vi "DestroyQ.vi"(8 "error in (no error)":errorcluster) -> (0 "error out":errorcluster)   [LabVIEW 2020, in "QDict.lvlib"]
doc: "Developed by Kevin Thompson\nkevin@thompsonengineering.net\n\nCopyright 2021\nThompson Engineering, LLC"
uses:
  QDict.lvlib
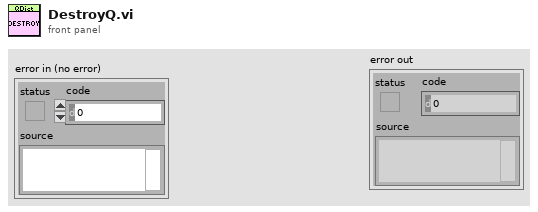
[diagram p1: front panel]
types:
  T1 = typedef "TD Dynamic CVT DVR--ref.ctl" = refnum<data-value>
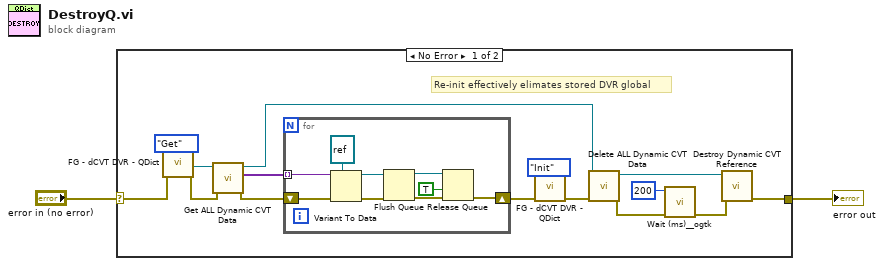
[diagram p0: block diagram]
diagram:
  n1 = case shown="No Error" "error in (no error)" {
    selector: "error in (no error)" -> [w16 w27]
    tunnel: [w3 w27] -> w2
    frame No Error {
      # "Re-init effectively elimates stored DVR global"
      n2 = call "FG - dCVT DVR - QDict.vi"("error in (no error)"=w16, "Action (Get)"=enum16{"Init", "Get", "Set"}."Get") -> ("dCVT QMH out"=w15:T1, "error out"=w14:errorcluster)  [unwired: 7 in]
      n3 = call <vilib>:"Get ALL Dynamic CVT Data.vi"("error in (no error)"=w14, "dCVT DVR"=w15) -> ("error out"=w13:errorcluster, "ValueArray"=w12:variant[], "dCVT DVR out"=w6:T1)  [unwired: 6 in, 1 out]
      n4 = for {
        shift-right: [w18] -> w8
        shift-left: w13 -> [w26]
        tunnel: w12 -> [w25] mode=indexing
        n5 = Variant To Data(error in=w26, type=refnum<queue> refnum ("queue out"), Variant=w25) -> (data=w22:refnum<queue>, error out=w23:errorcluster)
        n6 = Flush Queue(queue=w22, error in (no error)=w23) -> (queue out=w20:refnum<queue>, error out=w21:errorcluster)  [unwired: 1 out]
        n7 = Release Queue(queue=w20, force destroy? (F)=TRUE, error in (no error)=w21) -> (error out=w18:errorcluster)  [unwired: 2 out]
      }
      n8 = call "FG - dCVT DVR - QDict.vi"("error in (no error)"=w8, "Action (Get)"=enum16{"Init", "Get", "Set"}."Init") -> ("error out"=w7:errorcluster)  [unwired: 7 in, 1 out]
      n9 = call <vilib>:"Delete ALL Dynamic CVT Data.vi"("error in (no error)"=w7, "dCVT DVR"=w6) -> ("error out"=w10:errorcluster, "dCVT DVR out"=w5:T1)  [unwired: 8 in]
      n10 = call <userlib>:"Wait (ms)__ogtk.vi"("error in (no error)"=w10, "milliseconds to wait"=u32 200) -> ("error out"=w4:errorcluster)  [unwired: 8 in, 1 out]
      n11 = call <vilib>:"Destroy Dynamic CVT Reference.vi"("error in (no error)"=w4, "dCVT DVR"=w5) -> ("error out"=w3:errorcluster)  [unwired: 8 in, 1 out]
    }
    frame Error {
    }
  }
  "error out" <- w2
